vi "Tank_Burst_Strain.vi"() -> ()   [LabVIEW 2018]
uses:
  cluster_enum.ctl
  <vilib>/Utility/error.llb/DialogType.ctl
  <vilib>/DAQmx/read.llb/DAQmx Read (Analog 1D Wfm NChan NSamp).vi
  <vilib>/Waveform/WDTOps.llb/WDT Get Waveform Time Array DBL.vi
  <vilib>/DAQmx/configure/timing.llb/DAQmx Timing (Sample Clock).vi
  <vilib>/DAQmx/miscellaneous.llb/DAQmx Fill In Error Info.vi
  <resource>/objmgr/daqmx.rc
panel:
  in  "Tab Control":enum32{"Telemetry", "DAQ Settings"}(tab)
  in  "Stop 4":bool caption="Stop"
  out "Save Path":path caption="Path"
  in  "Test Name":string caption="String"
  in  "Save 2":bool caption="Save"
  in  "Strain Card 1 Tare":bool caption="Reset"
  in  "Strain Card 2 Tare":bool caption="Reset"
  in  "Strain Card 1 Rate Setpoint":dbl=1000.0 caption="Numeric"
  out "Strain Card 1 Rate":dbl caption="Numeric"
  in  "Strain Card 2 Rate Setpoint":dbl=100.0 caption="Numeric"
  out "Strain Card 2 Rate":dbl caption="Numeric"
  in  "Strain Card 1 Samples Per Loop":i32=100 caption="Numeric"
  in  "Strain Card 2 Samples Per Loop":i32=100 caption="Numeric"
  out "Strain Card 1":waveform(dbl)[](graph) caption="Waveform Chart"
  out "Strain Card 2":waveform(dbl)[](graph) caption="Waveform Chart"
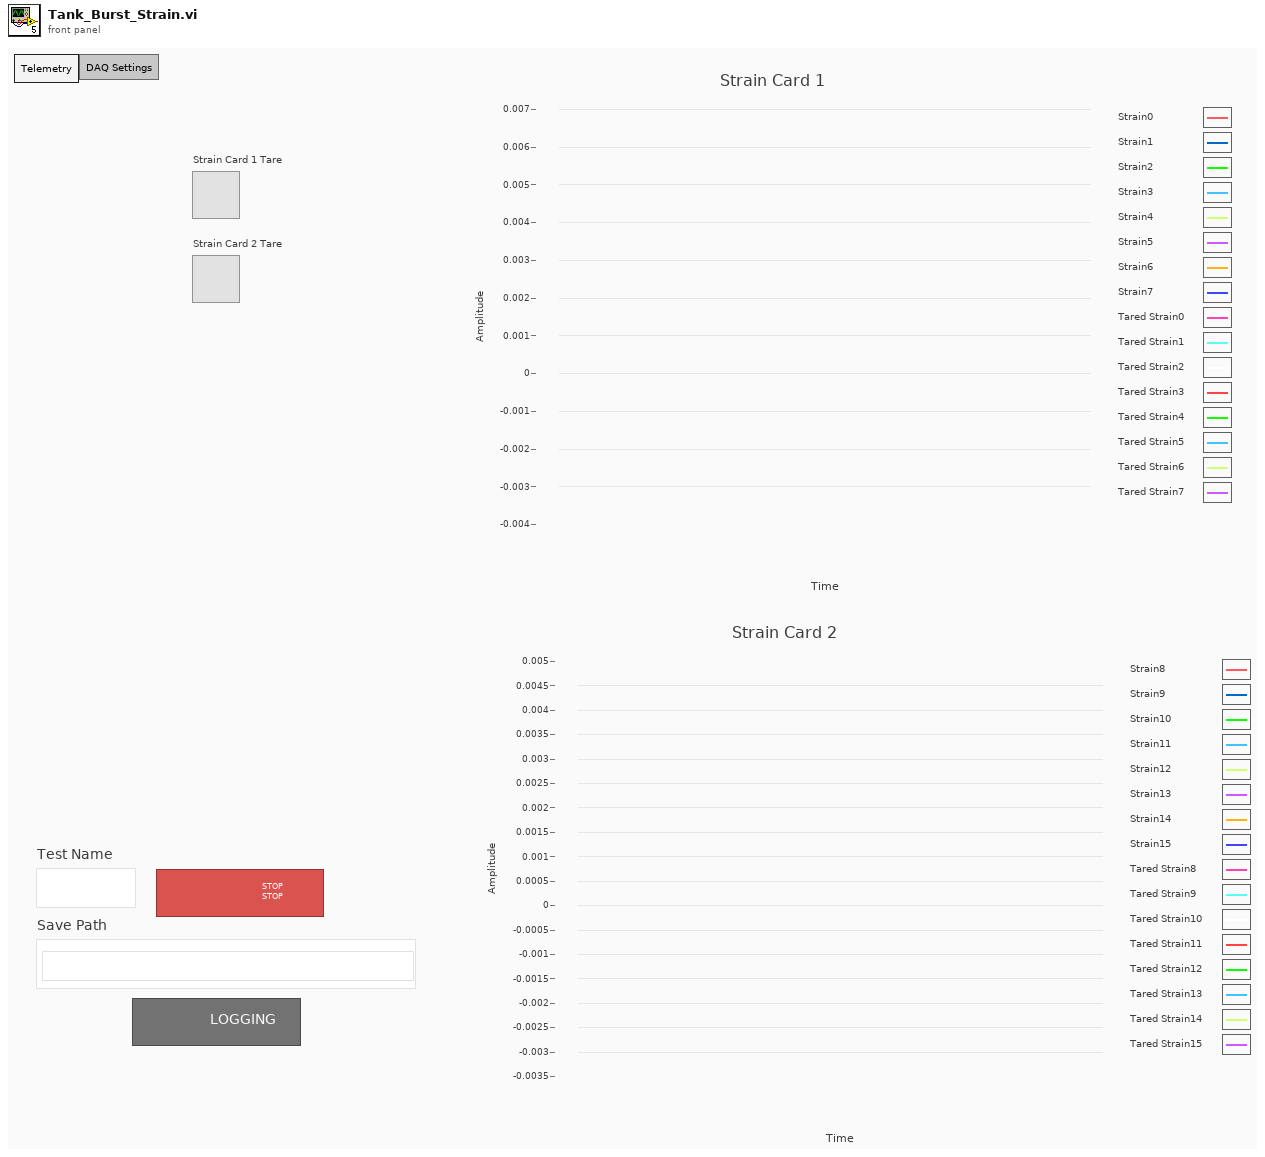
[diagram p1: front panel]
types:
  T1 = typedef "DialogType.ctl" = u16
  T2 = enum16{"open", "open or create", "create or replace", "create", "open (read-only)"}
  T3 = typedef "cluster_enum.ctl" = enum16{"Strain Card 2", "Strain Card 2 Tared", "Strain Card 1 Tared", "Strain Card 1"}
  T4 = cluster{"Strain Card":T3, "Strain Data":waveform(dbl)[]}
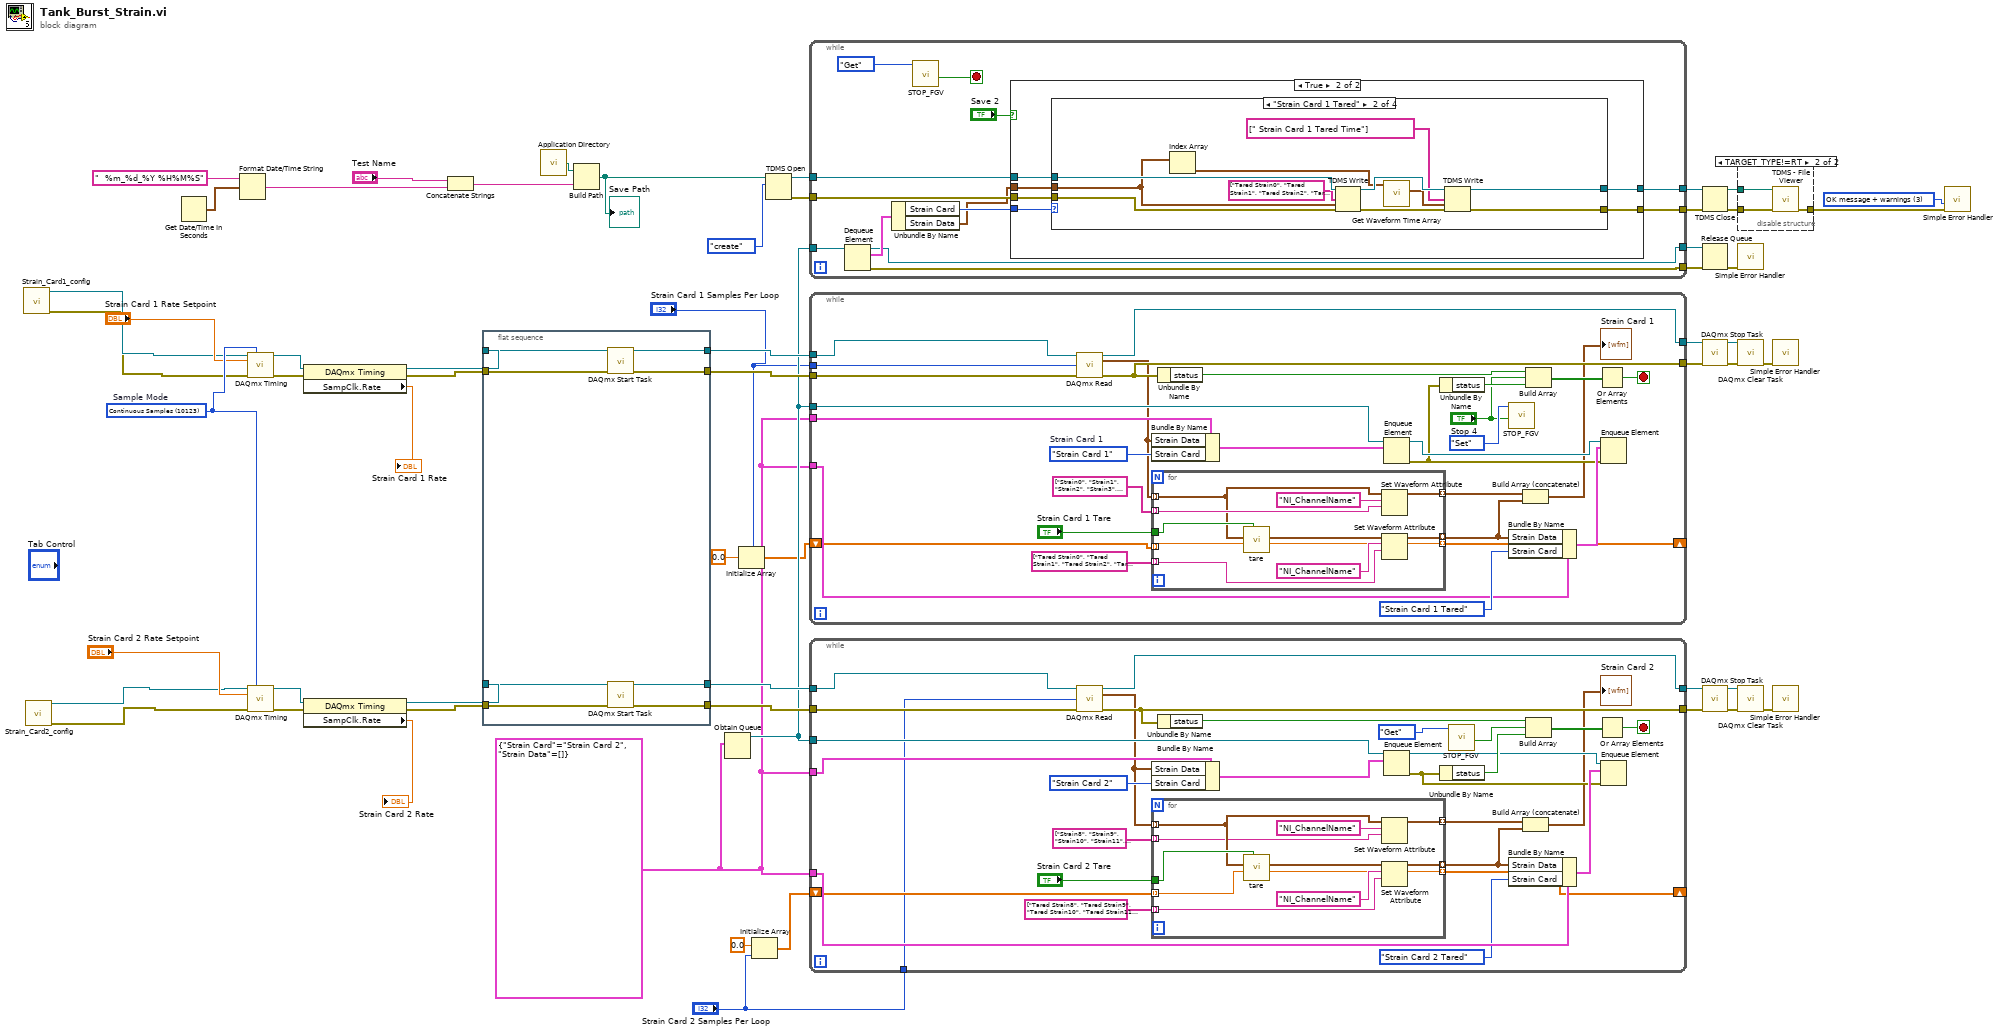
[diagram p0: block diagram]
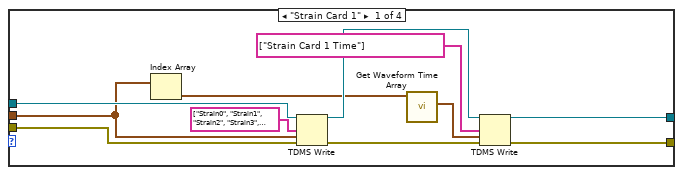
[diagram p4: hidden frame]
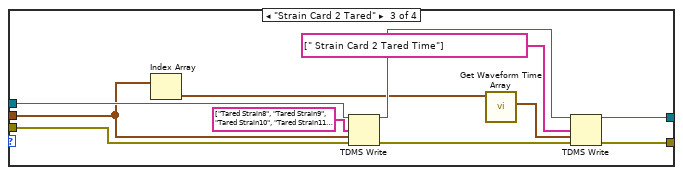
[diagram p5: hidden frame]
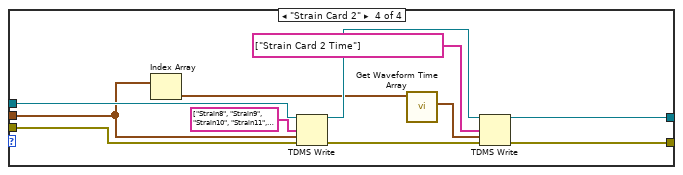
[diagram p6: hidden frame]
diagram:
  w20 = T1 3 items=["no dialog", "OK message", "continue or stop message", "OK message + warnings", "continue/stop + warnings"] ("type of dialog (OK msg:1)")
  w14 = T4 {"Strain Card"=enum."Strain Card 2", "Strain Data"=[]}
  w54 = 10123 items=["Finite Samples"=10178, "Continuous Samples"=10123, "Hardware Timed Single Point"=12522]  # Sample Mode
  n1 = call "Strain_Card1_config.vi"() -> ("error out"=w3:errorcluster, "task out"=w4:refnum<k21>)  [unwired: 10 in]
  n2 = call "Strain_Card2_config.vi"() -> ("error out"=w1:errorcluster, "task out"=w2:refnum<k21>)  [unwired: 10 in]
  n3 = Get Date/Time In Seconds() -> (seconds since 1Jan1904=w30:timestamp)
  n4 = Format Date/Time String(time format string (%c)="  %m_%d_%Y %H%M%S", seconds (now)=w30) -> (date/time string=w27:string)  [unwired: 1 in]
  n5 = call-poly <vilib>:"DAQmx Timing.vi"("task/channels in"=w4, "sample mode"=w54, "rate"="Strain Card 1 Rate Setpoint", "error in"=w3) -> ("task out"=w58:refnum<k21>, "error out"=w57:errorcluster)  [unwired: 10 in]
  n6 = call-poly <vilib>:"DAQmx Timing.vi"("task/channels in"=w2, "sample mode"=w54, "rate"="Strain Card 2 Rate Setpoint", "error in"=w1) -> ("task out"=w53:refnum<k21>, "error out"=w52:errorcluster)  [unwired: 10 in]
  n7 = property class="DAQmx Timing"(reference=w58, error in=w57) -> (reference out=w56:refnum<k21>, error out=w55:errorcluster, "SampClk.Rate"=→"Strain Card 1 Rate":dbl)
  n8 = property class="DAQmx Timing"(reference=w53, error in=w52) -> (reference out=w51:refnum<k21>, error out=w50:errorcluster, "SampClk.Rate"=→"Strain Card 2 Rate":dbl)
  n9 = Concatenate Strings("Test Name", w27) -> (w26:string)
  n10 = flat-sequence {
    tunnel: [w66] -> w45
    tunnel: w56 -> [w65]
    tunnel: w55 -> [w64]
    tunnel: [w63] -> w44
    tunnel: w51 -> [w62]
    tunnel: [w61] -> w32
    tunnel: [w60] -> w33
    tunnel: w50 -> [w59]
    frame #0 {
      n11 = call <vilib>:"DAQmx Start Task.vi"("task/channels in"=w65, "error in"=w64) -> ("task out"=w66:refnum<k21>, "error out"=w63:errorcluster)  [unwired: 12 in]
      n12 = call <vilib>:"DAQmx Start Task.vi"("task/channels in"=w62, "error in"=w59) -> ("task out"=w60:refnum<k21>, "error out"=w61:errorcluster)  [unwired: 12 in]
    }
  }
  n13 = call <vilib>:"Application Directory.vi"() -> ("Application Directory"=w28:path)
  n14 = Build Path(base path=w28, name or relative path=w26) -> (appended path=w25:path)
  "Save Path" <- w25
  n15 = Obtain Queue(element data type=w14) -> (queue out=w23:refnum<queue>)  [unwired: 4 in, 2 out]
  n16 = Initialize Array(0.0 ("element"), "Strain Card 1 Samples Per Loop") -> (w5:dbl[])
  n17 = Initialize Array(0.0 ("element"), "Strain Card 2 Samples Per Loop") -> (w8:dbl[])
  n18 = TDMS Open(10:T2."create" ("operation"), 11:w25) -> (0:w21:errorcluster, 3:w22:refnum<k34>)  [unwired: 5 in]
  n19 = while {
    tunnel: w23 -> [w79]
    tunnel: w22 -> [w76]
    tunnel: w21 -> [w75]
    tunnel: [w73] -> w16
    tunnel: [w72] -> w15
    tunnel: [w68] -> w12
    tunnel: [w67] -> w11
    stop <- w70 stop-if-true
    n20 = Dequeue Element(queue=w79) -> (queue out=w68:refnum<queue>, element=w78:T4, error out=w67:errorcluster)  [unwired: 2 in, 1 out]
    n21 = Unbundle By Name(w78) -> ("Strain Card"=w77:T3, "Strain Data"=w74:waveform(dbl)[])
    n22 = call "STOP_FGV.vi"("Mode"=enum16{"Set", "Get"}."Get") -> ("Get Value"=w70:bool)  [unwired: 9 in, 1 out]
    n23 = case shown="True" "Save 2" {
      tunnel: w77 -> [_ w87]
      tunnel: w76 -> [w81 w86]
      tunnel: w75 -> [w80 w85]
      tunnel: w74 -> [_ w84]
      tunnel: [w81 w83] -> w73
      tunnel: [w80 w82] -> w72
      frame False {
      }
      frame True {
        n24 = case shown="\"Strain Card 1 Tared\"" w87 {
          tunnel: w86 -> [w98 w109 w120 w131]
          tunnel: w85 -> [w97 w108 w119 w130]
          tunnel: w84 -> [w91 w102 w113 w124]
          tunnel: [w93 w104 w115 w126] -> w83
          tunnel: [w94 w105 w116 w127] -> w82
          frame "Strain Card 1" {
            n25 = Index Array(array=w91) -> (element=w90:waveform(dbl))  [unwired: 1 in]
            n26 = TDMS Write(0:w98, 7:string[] ["Strain0", "Strain1", "Strain2", "Strain3", "Strain4", "Strain5", "Strain6", "Strain7"] ("channel name(s) in (Untitled)"), 9:w91, 11:w97) -> (4:w96:refnum<k34>, 15:w95:errorcluster)  [unwired: 2 in, 2 out]
            n27 = call-poly <vilib>:"Get Waveform Time Array.vi"("waveform in"=w90) -> ("X array"=w89:timestamp[])  [unwired: 9 in, 1 out]
            n28 = TDMS Write(0:w96, 7:string[] ["Strain Card 1 Time"] ("channel name(s) in (Untitled)"), 9:w89, 11:w95) -> (4:w93:refnum<k34>, 15:w94:errorcluster)  [unwired: 2 in, 2 out]
          }
          frame "Strain Card 1 Tared" {
            n29 = Index Array(array=w102) -> (element=w101:waveform(dbl))  [unwired: 1 in]
            n30 = TDMS Write(0:w109, 7:string[] ["Tared Strain0", "Tared Strain1", "Tared Strain2", "Tared Strain3", "Tared Strain4", "Tared Strain5", "Tared Strain6", "Tared Strain7"] ("channel name(s) in (Untitled)"), 9:w102, 11:w108) -> (4:w107:refnum<k34>, 15:w106:errorcluster)  [unwired: 2 in, 2 out]
            n31 = call-poly <vilib>:"Get Waveform Time Array.vi"("waveform in"=w101) -> ("X array"=w100:timestamp[])  [unwired: 9 in, 1 out]
            n32 = TDMS Write(0:w107, 7:string[] [" Strain Card 1 Tared Time"] ("channel name(s) in (Untitled)"), 9:w100, 11:w106) -> (4:w104:refnum<k34>, 15:w105:errorcluster)  [unwired: 2 in, 2 out]
          }
          frame "Strain Card 2 Tared" {
            n33 = Index Array(array=w113) -> (element=w112:waveform(dbl))  [unwired: 1 in]
            n34 = TDMS Write(0:w120, 7:string[] ["Tared Strain8", "Tared Strain9", "Tared Strain10", "Tared Strain11", "Tared Strain12", "Tared Strain13", "Tared Strain14", "Tared Strain15"] ("channel name(s) in (Untitled)"), 9:w113, 11:w119) -> (4:w118:refnum<k34>, 15:w117:errorcluster)  [unwired: 2 in, 2 out]
            n35 = call-poly <vilib>:"Get Waveform Time Array.vi"("waveform in"=w112) -> ("X array"=w111:timestamp[])  [unwired: 9 in, 1 out]
            n36 = TDMS Write(0:w118, 7:string[] [" Strain Card 2 Tared Time"] ("channel name(s) in (Untitled)"), 9:w111, 11:w117) -> (4:w115:refnum<k34>, 15:w116:errorcluster)  [unwired: 2 in, 2 out]
          }
          frame "Strain Card 2" {
            n37 = Index Array(array=w124) -> (element=w123:waveform(dbl))  [unwired: 1 in]
            n38 = TDMS Write(0:w131, 7:string[] ["Strain8", "Strain9", "Strain10", "Strain11", "Strain12", "Strain13", "Strain14", "Strain15"] ("channel name(s) in (Untitled)"), 9:w124, 11:w130) -> (4:w129:refnum<k34>, 15:w128:errorcluster)  [unwired: 2 in, 2 out]
            n39 = call-poly <vilib>:"Get Waveform Time Array.vi"("waveform in"=w123) -> ("X array"=w122:timestamp[])  [unwired: 9 in, 1 out]
            n40 = TDMS Write(0:w129, 7:string[] ["Strain Card 2 Time"] ("channel name(s) in (Untitled)"), 9:w122, 11:w128) -> (4:w126:refnum<k34>, 15:w127:errorcluster)  [unwired: 2 in, 2 out]
          }
        }
      }
    }
  }
  n41 = while {
    tunnel: w45 -> [w156]
    tunnel: [w160] -> w41
    tunnel: w44 -> [w155]
    tunnel: [w153] -> w40
    tunnel: w23 -> [w149]
    tunnel: w14 -> [w152]
    tunnel: w14 -> [w146]
    tunnel: "Strain Card 1 Samples Per Loop" -> [w134]
    shift-right: [w132] -> _
    shift-left: w5 -> [w133]
    stop <- w159 stop-if-true
    w151 = cluster_enum."Strain Card 1"  # Strain Card 1
    n42 = call-poly <vilib>:"DAQmx Read.vi"("task/channels in"=w156, "number of samples per channel"=w134, "error in"=w155) -> ("task out"=w160:refnum<k21>, "data"=w139:waveform(dbl)[], "error out"=w153:errorcluster)  [unwired: 10 in]
    n43 = Bundle By Name(cluster=w152, "Strain Data"=w139, "Strain Card"=w151) -> (w150:T4)
    n44 = for {
      tunnel: w139 -> [w168] mode=indexing
      tunnel: [w163] -> w140 mode=indexing
      tunnel: "Strain Card 1 Tare" -> [w171]
      tunnel: string[] ["Strain0", "Strain1", "Strain2", "Strain3", "Strain4", "Strain5", "Strain6", "Strain7"] ("channel name(s) in (Untitled)") -> [w169] mode=indexing
      tunnel: [w167] -> w136 mode=indexing
      tunnel: string[] ["Tared Strain0", "Tared Strain1", "Tared Strain2", "Tared Strain3", "Tared Strain4", "Tared Strain5", "Tared Strain6", "Tared Strain7"] ("channel name(s) in (Untitled)") -> [w164] mode=indexing
      tunnel: w133 -> [w162] mode=indexing
      tunnel: [w161] -> w132 mode=indexing
      n45 = call "tare.vi"("Tare Control"=w171, "Shift Registor"=w162, "Input Waveform"=w168) -> ("Shift Registor Out"=w161:dbl, "output waveform"=w166:waveform(dbl))  [unwired: 7 in]
      n46 = Set Waveform Attribute(5:w169, 6:"NI_ChannelName" ("name"), 7:w168) -> (3:w167:waveform(dbl))  [unwired: 1 in, 2 out]
      n47 = Set Waveform Attribute(5:w164, 6:"NI_ChannelName" ("name"), 7:w166) -> (3:w163:waveform(dbl))  [unwired: 1 in, 2 out]
    }
    n48 = Unbundle By Name(w153) -> ("status"=w158:bool)
    n49 = Enqueue Element(queue=w149, element=w150) -> (queue out=w144:refnum<queue>, error out=w143:errorcluster)  [unwired: 2 in, 1 out]
    n50 = Unbundle By Name(w143) -> ("status"=w154:bool)
    n51 = call "STOP_FGV.vi"("Set Value"="Stop 4", "Mode"=enum16{"Set", "Get"}."Set") -> ()  [unwired: 8 in, 2 out]
    n52 = Bundle By Name(cluster=w146, "Strain Data"=w140, "Strain Card"=cluster_enum."Strain Card 1 Tared" ("Strain Card 1")) -> (w145:T4)
    n53 = Build Array (concatenate)(w136, w140) -> (→"Strain Card 1":waveform(dbl)[])
    n54 = Build Array(w158, "Stop 4", w154) -> (w157:bool[])
    n55 = Or Array Elements(Boolean array=w157) -> (logical OR=w159:bool)
    n56 = Enqueue Element(queue=w144, element=w145, error in (no error)=w143) -> ()  [unwired: 1 in, 3 out]
  }
  n57 = while {
    tunnel: w33 -> [w196]
    tunnel: [w200] -> w36
    tunnel: w32 -> [w195]
    tunnel: [w193] -> w35
    tunnel: w23 -> [w189]
    tunnel: w14 -> [w192]
    tunnel: w14 -> [w188]
    shift-right: [w174] -> _
    shift-left: w8 -> [w173]
    tunnel: "Strain Card 2 Samples Per Loop" -> [w172]
    stop <- w199 stop-if-true
    n58 = call-poly <vilib>:"DAQmx Read.vi"("task/channels in"=w196, "number of samples per channel"=w172, "error in"=w195) -> ("task out"=w200:refnum<k21>, "data"=w180:waveform(dbl)[], "error out"=w193:errorcluster)  [unwired: 10 in]
    n59 = Bundle By Name(cluster=w192, "Strain Data"=w180, "Strain Card"=cluster_enum."Strain Card 2" ("Strain Card 1")) -> (w190:T4)
    n60 = for {
      tunnel: w180 -> [w207] mode=indexing
      tunnel: [w210] -> w179 mode=indexing
      tunnel: "Strain Card 2 Tare" -> [w211]
      tunnel: string[] ["Tared Strain8", "Tared Strain9", "Tared Strain10", "Tared Strain11", "Tared Strain12", "Tared Strain13", "Tared Strain14", "Tared Strain15"] ("channel name(s) in (Untitled)") -> [w205] mode=indexing
      tunnel: string[] ["Strain8", "Strain9", "Strain10", "Strain11", "Strain12", "Strain13", "Strain14", "Strain15"] ("channel name(s) in (Untitled)") -> [w204] mode=indexing
      tunnel: [w206] -> w175 mode=indexing
      tunnel: [w202] -> w174 mode=indexing
      tunnel: w173 -> [w201] mode=indexing
      n61 = call "tare.vi"("Tare Control"=w211, "Shift Registor"=w201, "Input Waveform"=w207) -> ("Shift Registor Out"=w202:dbl, "output waveform"=w209:waveform(dbl))  [unwired: 7 in]
      n62 = Set Waveform Attribute(5:w204, 6:"NI_ChannelName" ("name"), 7:w207) -> (3:w206:waveform(dbl))  [unwired: 1 in, 2 out]
      n63 = Set Waveform Attribute(5:w205, 6:"NI_ChannelName" ("name"), 7:w209) -> (3:w210:waveform(dbl))  [unwired: 1 in, 2 out]
    }
    n64 = Unbundle By Name(w193) -> ("status"=w198:bool)
    n65 = Enqueue Element(queue=w189, element=w190) -> (queue out=w185:refnum<queue>, error out=w184:errorcluster)  [unwired: 2 in, 1 out]
    n66 = Unbundle By Name(w184) -> ("status"=w194:bool)
    n67 = call "STOP_FGV.vi"("Mode"=enum16{"Set", "Get"}."Get") -> ("Get Value"=w181:bool)  [unwired: 9 in, 1 out]
    n68 = Bundle By Name(cluster=w188, "Strain Data"=w179, "Strain Card"=cluster_enum."Strain Card 2 Tared" ("Strain Card 1")) -> (w186:T4)
    n69 = Build Array (concatenate)(w175, w179) -> (→"Strain Card 2":waveform(dbl)[])
    n70 = Build Array(w198, w181, w194) -> (w197:bool[])
    n71 = Or Array Elements(Boolean array=w197) -> (logical OR=w199:bool)
    n72 = Enqueue Element(queue=w185, element=w186, error in (no error)=w184) -> ()  [unwired: 1 in, 3 out]
  }
  n73 = TDMS Close(8:w15, 11:w16) -> (0:w18:errorcluster, 3:w19:path)
  n74 = Release Queue(queue=w12, error in (no error)=w11) -> (error out=w13:errorcluster)  [unwired: 1 in, 2 out]
  n75 = call <vilib>:"DAQmx Stop Task.vi"("task/channels in"=w41, "error in"=w40) -> ("task out"=w43:refnum<k21>, "error out"=w42:errorcluster)  [unwired: 12 in]
  n76 = call <vilib>:"DAQmx Stop Task.vi"("task/channels in"=w36, "error in"=w35) -> ("task out"=w38:refnum<k21>, "error out"=w37:errorcluster)  [unwired: 12 in]
  n77 = disable-structure shown="TARGET_TYPE!=RT" {
    disable-tunnel: w18 -> [w212 w215]
    disable-tunnel: w19 -> [_ w214]
    disable-tunnel: [w212 w213] -> w17
    frame condition #0 {
    }
    frame condition #1 (active) {
      n78 = call <vilib>:"TDMS - File Viewer.vi"("error in (no error)"=w215, "file path"=w214) -> ("error out"=w213:errorcluster)  [unwired: 5 out]
    }
  }
  n79 = call <vilib>:"Simple Error Handler.vi"("error in (no error)"=w13) -> ()  [unwired: 1 in, 8 out]
  n80 = call <vilib>:"DAQmx Clear Task.vi"("task in"=w43, "error in"=w42) -> ("error out"=w39:errorcluster)  [unwired: 13 in]
  n81 = call <vilib>:"DAQmx Clear Task.vi"("task in"=w38, "error in"=w37) -> ("error out"=w34:errorcluster)  [unwired: 13 in]
  n82 = call <vilib>:"Simple Error Handler.vi"("error in (no error)"=w39) -> ()  [unwired: 1 in, 8 out]
  n83 = call <vilib>:"Simple Error Handler.vi"("error in (no error)"=w34) -> ()  [unwired: 1 in, 8 out]
  n84 = call <vilib>:"Simple Error Handler.vi"("type of dialog (OK msg:1)"=w20, "error in (no error)"=w17) -> ()  [unwired: 1 in, 7 out]
